vi "Dispatch Measure Async.vi"(8 "error in (no error)":errorcluster, 9 "measurement plugin service in":refnum<class "Measurement Plugin Service.lvclass">, 10 "gRPC ID in":T1, 11 "measurement service in":refnum<class "IMeasurement Service.lvclass">) -> (0 "error out":errorcluster)   [LabVIEW 2021, in "NI Measurement Plug-In SDK.lvlib" / "IMeasurement Service.lvclass"]
uses:
  IMeasurement Service.lvclass
  <vilib>/gRPC/LabVIEW gRPC Library/Shared/grpcId.ctl
  Measurement Plugin Service/Measurement Plugin Service.lvclass
  Handle Measure RPC.vi
  <vilib>/gRPC/LabVIEW gRPC Library/grpc-lvsupport-release.lvlib
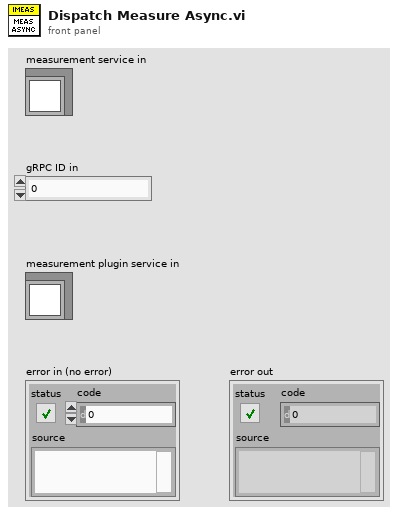
[diagram p1: front panel]
types:
  T1 = typedef "grpc-lvsupport-release.lvlib/grpcId.ctl" = u64
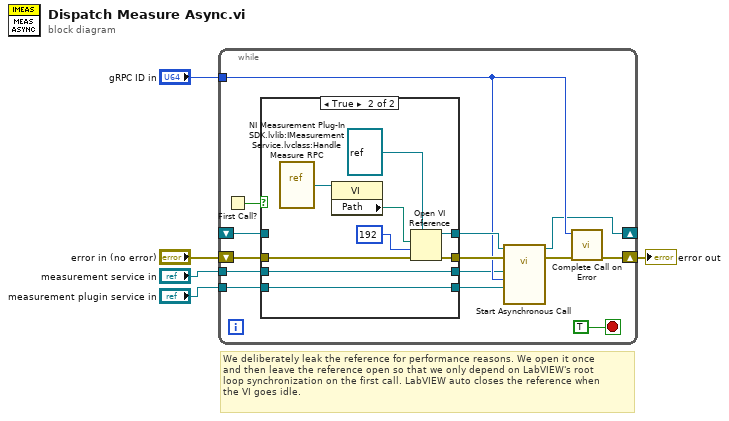
[diagram p0: block diagram]
diagram:
  # "We deliberately leak the reference for performance reasons. We open it once\nand then leave the reference open so that we only depend on LabVIEW's root\nloop synchronization on the first call. LabVIEW auto closes the reference when\nthe VI goes idle."
  n1 = while {
    tunnel: "gRPC ID in" -> [w15]
    tunnel: "measurement plugin service in" -> [w13]
    tunnel: "measurement service in" -> [w11]
    shift-right: [w16] -> w4
    shift-left: "error in (no error)" -> [w17]
    shift-right: [w6] -> _
    shift-left: _ -> [w7]
    stop <- TRUE stop-if-true
    n2 = First Call?() -> (First Call?: T/F=w14:bool)
    n3 = case shown="True" w14 {
      tunnel: [w20 w30] -> w19
      tunnel: [w23 w29] -> w18
      tunnel: w17 -> [w23 w28]
      tunnel: w13 -> [w22 w25]
      tunnel: [w22 w25] -> w12
      tunnel: w11 -> [w21 w24]
      tunnel: [w21 w24] -> w10
      tunnel: w7 -> [w20 _]
      frame False {
      }
      frame True {
        n4 = vi-ref "NI Measurement Plug-In SDK.lvlib:IMeasurement Service.lvclass:Handle Measure RPC.vi"() -> (w27:refnum<vi>)
        n5 = property class="VI"(reference=w27) -> ("Path"=w26:path)  [unwired: 1 in, 2 out]
        n6 = Open VI Reference(type specifier VI Refnum (for type only)=refnum<vi> refnum, vi path=w26, options=192, error in (no error)=w28) -> (vi reference=w30:refnum<vi>, error out=w29:errorcluster)  [unwired: 2 in]
      }
    }
    n7 = call-by-ref "Start Asynchronous Call"(reference=w19, error in=w18, "measurement plugin service in"=w12, "gRPC ID in"=w15, "measurement service in"=w10) -> (reference out=w6:refnum<vi>, error out=w9:errorcluster)  [unwired: 9 in]
    n8 = call "Complete Call on Error.vi"("error in"=w9, "gRPC ID in"=w15) -> ("error out"=w16:errorcluster)  [unwired: 9 in]
  }
  "error out" <- w4
